vi "GUI_telemetry.vi"() -> ()   [LabVIEW 2013]
uses:
  shared programs/GUI_Template/GUI_master/tcp_new_data_event.ctl
  shared programs/GUI_Template/GUI_master/tcp new data cluster.ctl
panel:
  in  "All On":bool
  in  "All Off":bool
  in  "Color Ch 15":u32(colorbox)=16740860
  in  "Color Ch 14":u32(colorbox)=14417753
  in  "Color Ch 13":u32(colorbox)=16741233
  in  "Color Ch 12":u32(colorbox)=7209097
  in  "Color Ch 11":u32(colorbox)=12105912
  in  "Color Ch 10":u32(colorbox)=16740772
  in  "Color Ch 9":u32(colorbox)=7470977
  in  "Color Ch 8":u32(colorbox)=35208
  in  "Color Ch 7":u32(colorbox)=16756736
  in  "Color Ch 6":u32(colorbox)=16711885
  in  "Color Ch 5":u32(colorbox)=56375
  in  "Color Ch 4":u32(colorbox)=9567230
  in  "Color Ch 3":u32(colorbox)=16776704
  in  "Color Ch 2":u32(colorbox)=16777225
  in  "Color Ch 1":u32(colorbox)=16711680
  in  "Color Ch 0":u32(colorbox)=4355583
  in  "On CH":bool[](array[boolean])
  in  "display 15":bool=TRUE
  in  "display 14":bool=TRUE
  in  "display 13":bool=TRUE
  in  "display 12":bool=TRUE
  in  "display 11":bool=TRUE
  in  "display 10":bool=TRUE
  in  "display 9":bool=TRUE
  in  "display 8":bool=TRUE
  in  "display 7":bool=TRUE
  in  "display 6":bool=TRUE
  in  "display 5":bool=TRUE
  in  "display 4":bool=TRUE
  in  "display 3":bool=TRUE
  in  "display 2":bool=TRUE
  in  "display 1":bool=TRUE
  in  "display 0":bool=TRUE
  out "Waveform Chart":T1(graph)
  in  "Reading.channel 14::1":dbl caption="Ch 14: Gamma CaveA ceiling #1" min=-10.0 max=1000.0 format="%.3f"
  in  "Reading.channel 13::1":dbl caption="Ch 13: Gamma CaveB ceiling #2" min=-10.0 max=1000.0 format="%.3f"
  in  "Reading.channel 15::1":dbl caption="Ch 15: Gamma Cavea ceiling #2" min=-10.0 max=1000.0 format="%.3f"
  in  "Reading.channel 3::1":dbl caption="Ch 3: 10TW Gamma [far]" min=-10.0 max=1000.0 format="%.3f"
  in  "Reading.channel 2::1":dbl caption="Ch 2: 10TW Gamma [near]" min=-10.0 max=1000.0 format="%.3f"
  in  "Reading.channel 1::1":dbl caption="Ch 1: 10TW Rep Rate" min=-10.0 max=1000.0 format="%.3f"
  in  "Reading.channel 0::1":dbl caption="Ch 0: 10TW Neutron" min=-10.0 max=1000.0 format="%.3f"
  in  "Reading.channel 12::1":dbl caption="Ch 12: Gamma CaveB ceiling #1" min=-10.0 max=1000.0 format="%.3f"
  in  "Reading.channel 11::1":dbl caption="Ch 11: Staged Neutron" min=-10.0 max=1000.0 format="%.3f"
  in  "Reading.channel 4::1":dbl caption="Ch 4: 100TW Gamma [near]" min=-10.0 max=1000.0 format="%.3f"
  in  "Reading.channel 5::1":dbl caption="Ch 5: 100TW Gamma [far]" min=-10.0 max=1000.0 format="%.3f"
  in  "Reading.channel 6::1":dbl caption="Ch 6: Gamma Cave-B Roof" min=-10.0 max=1000.0 format="%.3f"
  in  "Reading.channel 7::1":dbl caption="Ch 7: Gamma behind Cave-A" min=-10.0 max=1000.0 format="%.3f"
  in  "Reading.channel 9::1":dbl caption="Ch 9: 100TW Rep Rate" min=-10.0 max=1000.0 format="%.3f"
  in  "Reading.channel 8::1":dbl caption="Ch 8: 100TW Neutron" min=-10.0 max=1000.0 format="%.3f"
  in  "Reading.channel 10::1":dbl caption="Ch 10: Staged Gamma" min=-10.0 max=1000.0 format="%.3f"
  in  "GUIdevice 1":string="RadiationTelemetry"
  in  "insert tag":bool=TRUE
  in  "stop":bool
  out "tcp data event":T2
  out "error IO 2":errorcluster
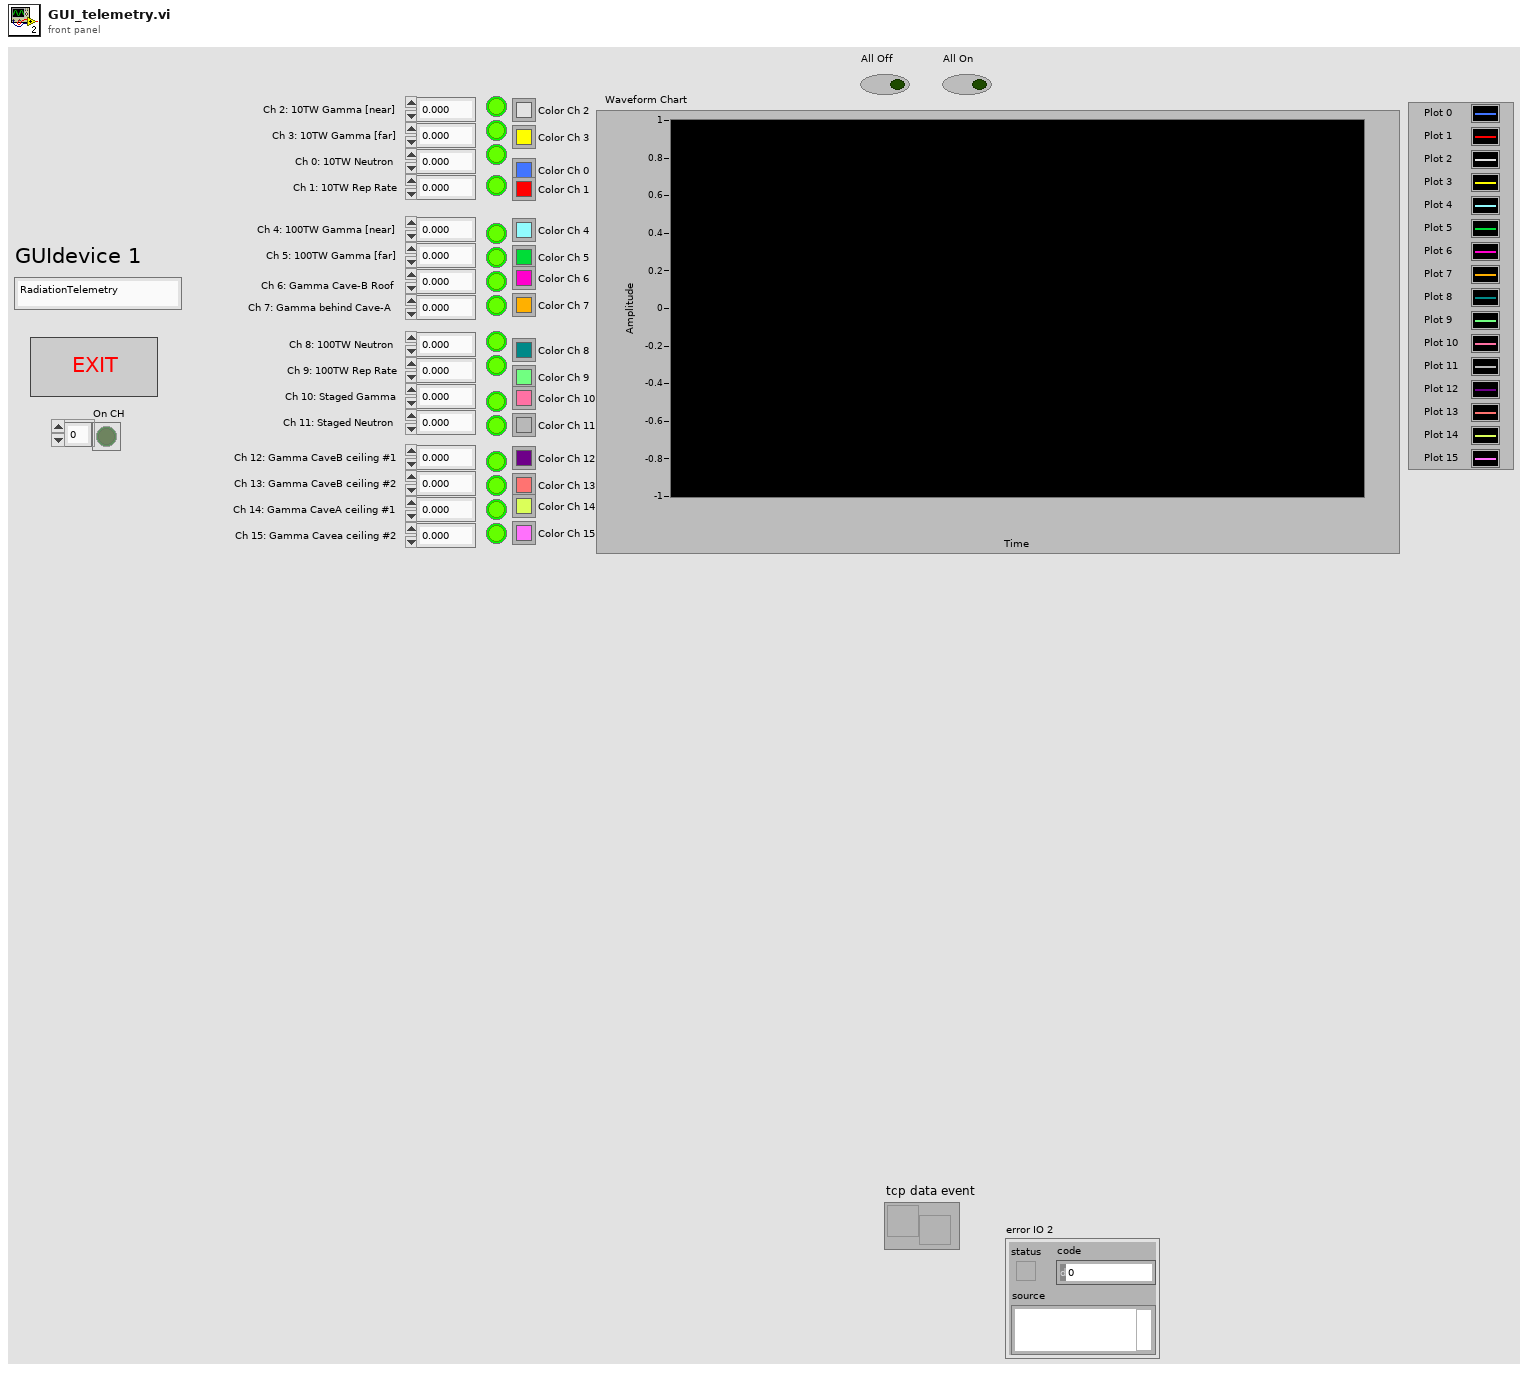
[diagram p1: front panel]
types:
  T1 = cluster{"Reading.channel 0::1":dbl, "Reading.channel 1::1":dbl, "Reading.channel 2::1":dbl, "Reading.channel 3::1":dbl, "Reading.channel 4::1":dbl, "Reading.channel 5::1":dbl, "Reading.channel 6::1":dbl, "Reading.channel 7::1":dbl, "Reading.channel 8::1":dbl, "Reading.channel 9::1":dbl, "Reading.channel 10::1":dbl, "Reading.channel 11::1":dbl, "Reading.channel 12::1":dbl, "Reading.channel 13::1":dbl, "Reading.channel 14::1":dbl, "Reading.channel 15::1":dbl}
  T2 = typedef "tcp_new_data_event.ctl" = refnum<user-event>
  T3 = typedef "tcp new data cluster.ctl" = cluster{"EventEnum":enum16{"new data", "connection status update"}, "Device name":string}
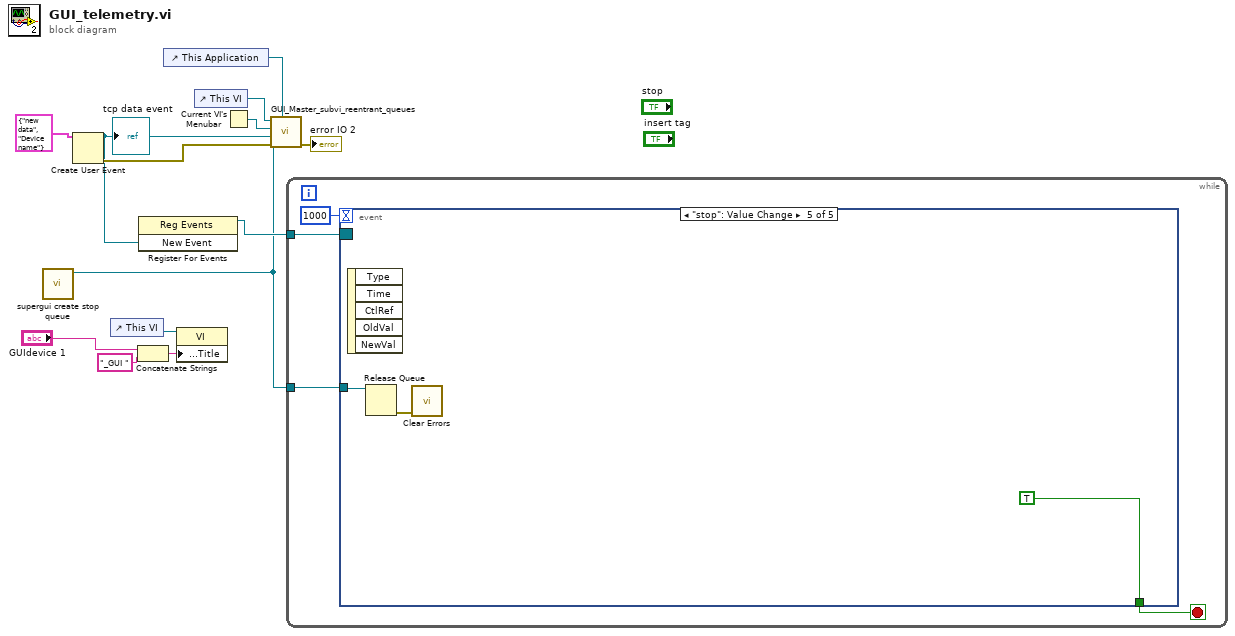
[diagram p0: block diagram]
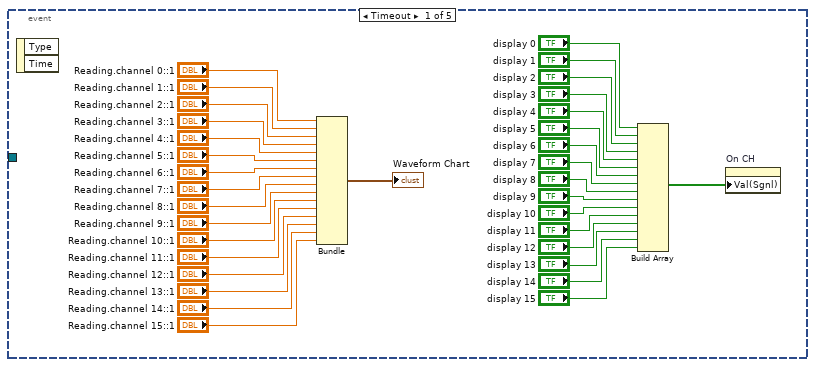
[diagram p2: hidden frame]
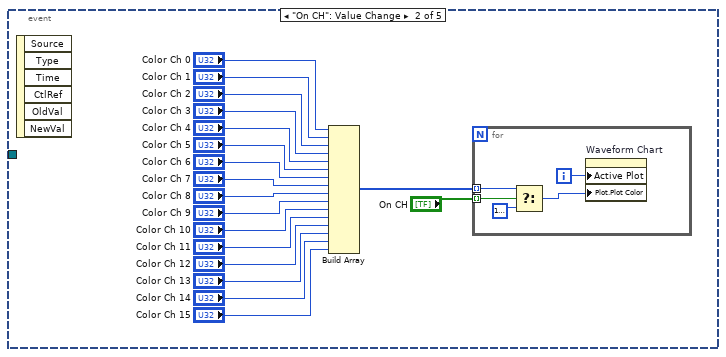
[diagram p3: hidden frame]
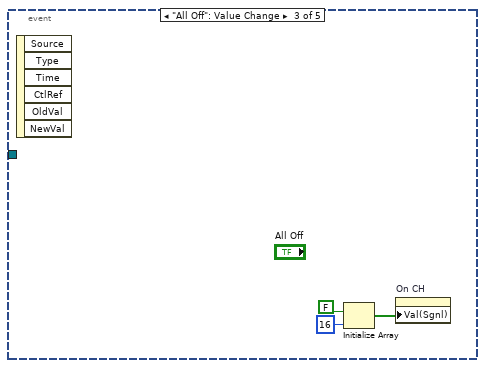
[diagram p4: hidden frame]
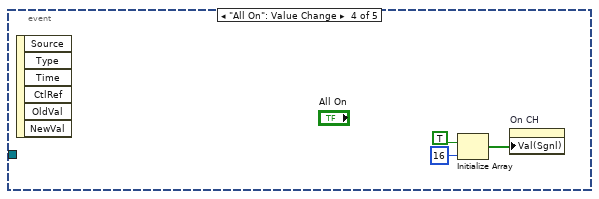
[diagram p5: hidden frame]
diagram:
  n1 = call "supergui create stop queue.vi"() -> ("STOP Queue out"=w5:refnum<queue>)  [unwired: 11 in]
  n2 = Create User Event(user event datatype=T3 {"EventEnum"=enum."new data", "Device name"="Device name"} ("New Event")) -> (user event=w7:refnum<user-event>, error out=w9:errorcluster)  [unwired: 1 in]
  "tcp data event" <- w7
  n3 = control-ref of="This VI"() -> (w4:refnum<vi>)
  n4 = Concatenate Strings("GUIdevice 1", "_GUI ") -> (w3:string)
  n5 = register-events(w7) -> (reference out=w6:refnum<event-registration>)  [unwired: 2 in, 1 out]
  n6 = control-ref of="This Application"() -> (w8:refnum<vi>)
  n7 = property class="VI"(reference=w4, "Front Panel.Title"=w3) -> ()  [unwired: 1 in, 2 out]
  n8 = control-ref of="This VI"() -> (w12:refnum<vi>)
  n9 = Current VI's Menubar() -> (w11:refnum<k9>)
  n10 = call "GUI_Master_subvi_reentrant_queues.vi"("STOP Queue in"=w5, "This Application"=w8, "error in (no error)"=w9, "tcp data event"=w7, "Caller menu reference"=w11, "Caller VI ref"=w12) -> ("error out"=→"error IO 2":errorcluster)  [unwired: 5 in]
  n11 = while {
    tunnel: w6 -> [w16]
    tunnel: w5 -> [w14]
    stop <- w17 stop-if-true
    n12 = event shown="[4] \"stop\": Value Change" {
      selector: w16 -> [_ _ _ _ _]
      dyn-events: _ -> [_ _ _ _ _]
      timeout: 1000 -> [_ _ _ _ _]
      tunnel: [_ _ _ _ TRUE] -> w17
      tunnel: w14 -> [_ _ _ _ w82]
      event Timeout {
        n13 = event-data() -> ()  [unwired: 1 in, 2 out]
        n14 = Bundle("Reading.channel 0::1"="Reading.channel 0::1", "Reading.channel 1::1"="Reading.channel 1::1", "Reading.channel 2::1"="Reading.channel 2::1", "Reading.channel 3::1"="Reading.channel 3::1", "Reading.channel 4::1"="Reading.channel 4::1", "Reading.channel 5::1"="Reading.channel 5::1", "Reading.channel 6::1"="Reading.channel 6::1", "Reading.channel 7::1"="Reading.channel 7::1", "Reading.channel 8::1"="Reading.channel 8::1", "Reading.channel 9::1"="Reading.channel 9::1", "Reading.channel 10::1"="Reading.channel 10::1", "Reading.channel 11::1"="Reading.channel 11::1", "Reading.channel 12::1"="Reading.channel 12::1", "Reading.channel 13::1"="Reading.channel 13::1", "Reading.channel 14::1"="Reading.channel 14::1", "Reading.channel 15::1"="Reading.channel 15::1") -> (→"Waveform Chart":T1)  [unwired: 1 in]
        n15 = Build Array("display 0", "display 1", "display 2", "display 3", "display 4", "display 5", "display 6", "display 7", "display 8", "display 9", "display 10", "display 11", "display 12", "display 13", "display 14", "display 15") -> (w18:bool[])
        n16 = property on="On CH" class="Arr (strict)"("Val(Sgnl)"=w18) -> ()  [unwired: 2 in, 2 out]
      }
      event "On CH": Value Change {
        n17 = event-data() -> ()  [unwired: 1 in, 6 out]
        n18 = Build Array("Color Ch 0", "Color Ch 1", "Color Ch 2", "Color Ch 3", "Color Ch 4", "Color Ch 5", "Color Ch 6", "Color Ch 7", "Color Ch 8", "Color Ch 9", "Color Ch 10", "Color Ch 11", "Color Ch 12", "Color Ch 13", "Color Ch 14", "Color Ch 15") -> (w53:u32[])
        n19 = for {
          tunnel: "On CH" -> [w73] mode=indexing
          tunnel: w53 -> [w70] mode=indexing
          i -> [w74]
          n20 = Select(t=w70, s=w73, f=u32 16777216 ("Color Ch 0")) -> (s? t:f=w72:u32)
          n21 = property on="Waveform Chart" class="WFChart (strict)"("Active Plot"=w74, "Plot.Plot Color"=w72) -> ()  [unwired: 2 in, 2 out]
        }
      }
      event "All Off": Value Change {
        n22 = event-data() -> ()  [unwired: 1 in, 6 out]
        n23 = Initialize Array(FALSE, 16 ("dimension size")) -> (w75:bool[])
        n24 = property on="On CH" class="Arr (strict)"("Val(Sgnl)"=w75) -> ()  [unwired: 2 in, 2 out]
      }
      event "All On": Value Change {
        n25 = event-data() -> ()  [unwired: 1 in, 6 out]
        n26 = Initialize Array(TRUE, 16 ("dimension size")) -> (w78:bool[])
        n27 = property on="On CH" class="Arr (strict)"("Val(Sgnl)"=w78) -> ()  [unwired: 2 in, 2 out]
      }
      event "stop": Value Change {
        n28 = event-data() -> ()  [unwired: 1 in, 5 out]
        n29 = Release Queue(queue=w82) -> (error out=w81:errorcluster)  [unwired: 2 in, 2 out]
        n30 = call <vilib>:"Clear Errors.vi"("error in (no error)"=w81) -> ()  [unwired: 6 in, 1 out]
      }
    }
  }
